vi "AbsMinMax(subVi).vi"(8 "y":dbl, 11 "x":dbl) -> (0 "abs min":dbl, 3 "abs max":dbl)   [LabVIEW 2021]
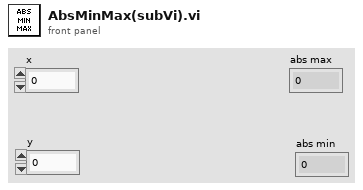
[diagram p1: front panel]
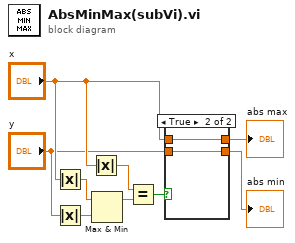
[diagram p0: block diagram]
diagram:
  n1 = Absolute Value(x="x") -> (abs(x)=w9:dbl)
  n2 = Absolute Value(x="y") -> (abs(x)=w8:dbl)
  n3 = Absolute Value(x="x") -> (abs(x)=w7:dbl)
  n4 = Max & Min(x=w9, y=w8) -> (max(x,y)=w6:dbl)  [unwired: 1 out]
  n5 = Equal?(x=w7, y=w6) -> (x = y?=w5:bool)
  n6 = case shown="True" w5 {
    tunnel: [w11 w13] -> w4
    tunnel: "x" -> [w10 w13]
    tunnel: "y" -> [w11 w12]
    tunnel: [w10 w12] -> w1
    frame False {
    }
    frame True {
    }
  }
  "abs max" <- w4
  "abs min" <- w1
